vi "angular velocity.vi"() -> ()   [LabVIEW 2009]
uses:
  <vilib>/DAQmx/create/channels.llb/DAQmx Create Channel (CI-Position-Angular Encoder).vi
  <vilib>/DAQmx/read.llb/DAQmx Read (Counter DBL 1Chan 1Samp).vi
panel:
  out "Position Graph":dbl[](graph)
  out "Velocity Graph":dbl[](graph)
  in  "Decoding Type":i32(ring)=10092 items=["X1"=10090, "X2"=10091, "X4"=10092, "Two Pulse Counting"=10313]
  in  "Pulses per Revolution":u32=24
  in  "Z Index Phase":i32(ring)=10040 items=["A High B High"=10040, "A High B Low"=10041, "A Low B High"=10042, "A Low B Low"=10043]
  in  "Z Index Value":dbl
  in  "Z Index Enable":bool
  in  "Counter(s)":tag="Dev1/ctr0" caption="Counter"
  in  "stop":bool
  out "Velocity":dbl
  out "Position":dbl
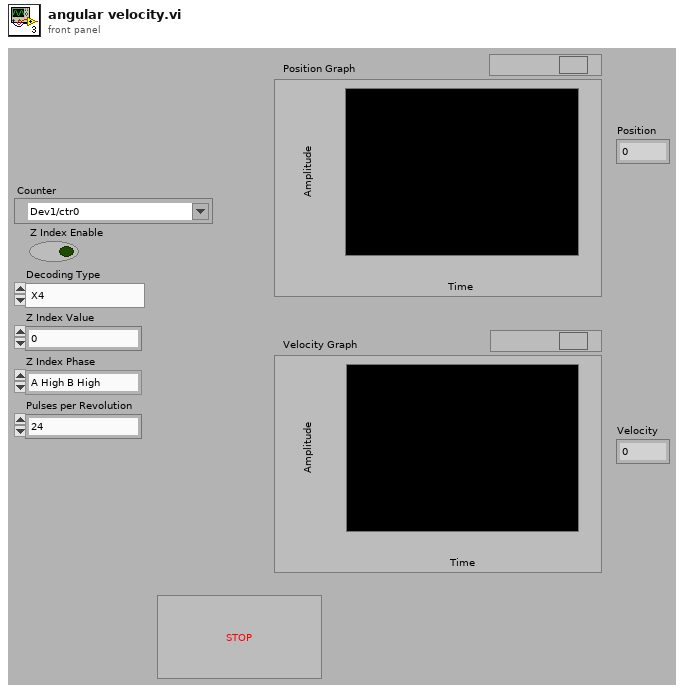
[diagram p1: front panel]
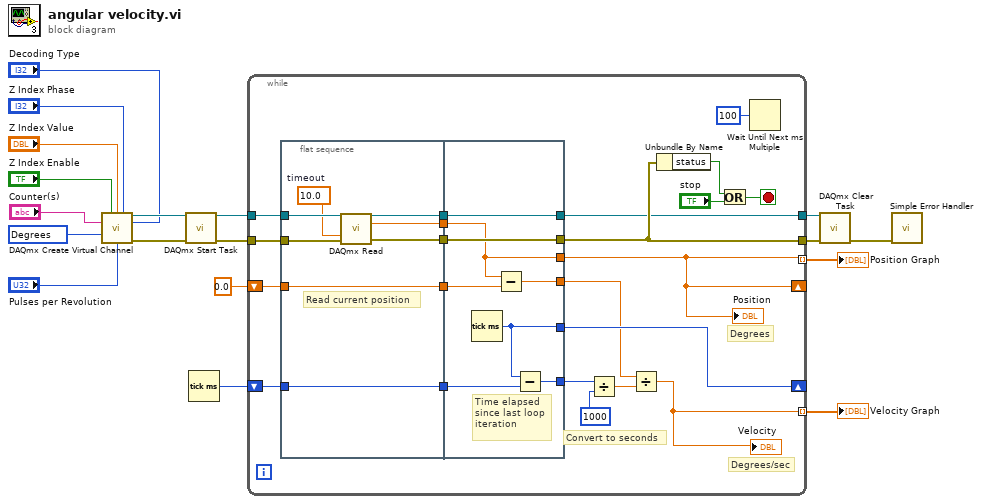
[diagram p0: block diagram]
diagram:
  w5 = 10146 items=["Degrees"=10146, "Radians"=10273, "Ticks"=10304, "From Custom Scale"=10065] ("units")
  n1 = call-poly <vilib>:"DAQmx Create Virtual Channel.vi"("z index enable"="Z Index Enable", "z index value"="Z Index Value", "z index phase"="Z Index Phase", "counter"="Counter(s)", "decoding type"="Decoding Type", "units"=w5, "pulses per revolution"="Pulses per Revolution") -> ("task out"=w14:refnum<k21>, "error out"=w2:errorcluster)  [unwired: 7 in]
  n2 = call <vilib>:"DAQmx Start Task.vi"("task/channels in"=w14, "error in"=w2) -> ("task out"=w16:refnum<k21>, "error out"=w4:errorcluster)  [unwired: 12 in]
  n3 = Tick Count (ms)() -> (millisecond timer value=w7:u32)
  n4 = while {
    tunnel: w4 -> [w40]
    tunnel: [w36] -> w18
    tunnel: w16 -> [w35]
    tunnel: [w34] -> w15
    shift-right: [w30] -> _
    shift-left: w7 -> [w21]
    shift-right: [w19] -> _
    shift-left: 0.0 ("data") -> [w27]
    tunnel: [w25] -> w3 mode=indexing
    tunnel: [w19] -> w1 mode=indexing
    stop <- w39 stop-if-true
    # "Degrees"
    # "Degrees/sec"
    # "Convert to seconds"
    n5 = flat-sequence {
      tunnel: w40 -> [w48]
      tunnel: w35 -> [w46]
      tunnel: [w47] -> w32
      tunnel: [w45] -> w31
      tunnel: [w43] -> w29
      tunnel: [w42] -> w28
      tunnel: w27 -> [w42]
      tunnel: w21 -> [w41]
      tunnel: [w41] -> w20
      tunnel: [w55] -> w34
      tunnel: [w56] -> w36
      tunnel: w32 -> [w56]
      tunnel: w31 -> [w55]
      tunnel: [w50] -> w30
      tunnel: w29 -> [w52]
      tunnel: w28 -> [w51]
      tunnel: [w54] -> w26
      tunnel: [w52] -> w19
      tunnel: [w53] -> w24
      tunnel: w20 -> [w49]
      frame #0 {
        w44 = 10.0  # timeout
        # "Read current position"
        n6 = call-poly <vilib>:"DAQmx Read.vi"("task/channels in"=w46, "timeout"=w44, "error in"=w48) -> ("task out"=w45:refnum<k21>, "data"=w43:dbl, "error out"=w47:errorcluster)  [unwired: 10 in]
      }
      frame #1 {
        # "Time elapsed \nsince last loop\niteration"
        n7 = Tick Count (ms)() -> (millisecond timer value=w50:u32)
        n8 = Subtract(x=w52, y=w51) -> (x-y=w54:dbl)
        n9 = Subtract(x=w50, y=w49) -> (x-y=w53:u32)
      }
    }
    n10 = Divide(x=w24, y=u32 1000) -> (x/y=w22:dbl)
    n11 = Divide(x=w26, y=w22) -> (x/y=w25:dbl)
    "Velocity" <- w25
    n12 = Unbundle By Name(w36) -> ("status"=w37:bool)
    n13 = Or(x=w37, y="stop") -> (x .or. y?=w39:bool)
    n14 = Wait Until Next ms Multiple(millisecond multiple=u32 100) -> ()  [unwired: 1 out]
    "Position" <- w19
  }
  "Velocity Graph" <- w3
  "Position Graph" <- w1
  n15 = call <vilib>:"DAQmx Clear Task.vi"("task in"=w15, "error in"=w18) -> ("error out"=w17:errorcluster)  [unwired: 13 in]
  n16 = call <vilib>:"Simple Error Handler.vi"("error in (no error)"=w17) -> ()  [unwired: 4 in, 5 out]
